vi "Reset Device Core.vi"(8 "error in (no error)":errorcluster, 11 "LS218 in":refnum<class "LS218.lvclass">) -> (0 "error out":errorcluster, 3 "LS218 out":refnum<class "LS218.lvclass">)   [LabVIEW 2013, in "LS218.lvlib" / "LS218.lvclass"]
doc: "Perform reset of device."
uses:
  LS218.lvclass
  CSPP_Core/Actors/CS++DeviceActor/CS++DeviceActor.lvclass
  CSPP_Core/Actors/CS++DeviceActor/CS++DeviceActor.lvclass/CS++DeviceActor.ctl
  LS218.lvclass/LS218.ctl
  CSPP_Core/Actors/CS++DeviceActor/Read ResetWithDefaults.vi
  <instrlib>/Lake Shore Cryotronics 218/Lake Shore Cryotronics 218.lvlib
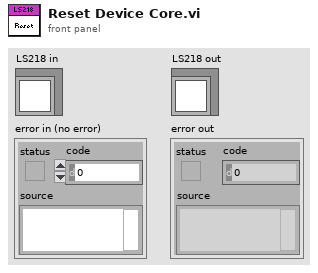
[diagram p1: front panel]
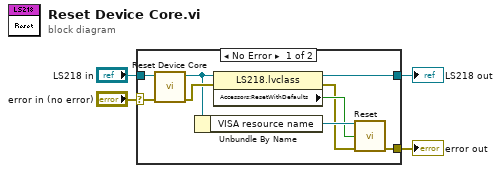
[diagram p0: block diagram]
diagram:
  n1 = case shown="No Error" "error in (no error)" {
    selector: "error in (no error)" -> [w5 w14]
    tunnel: "LS218 in" -> [w13 w15]
    tunnel: [w10 w15] -> w3
    tunnel: [w6 w14] -> w2
    frame No Error {
      n2 = call-parent "Reset Device Core.vi"("error in (no error)"=w5, "CS++DeviceActor in"=w13) -> ("error out"=w9:errorcluster, "CS++DeviceActor out"=w8:refnum<class "LS218.lvclass">)  [unwired: 8 in]
      n3 = Unbundle By Name(w8) -> ("VISA resource name"=w12:refnum<visa-resource-name>)
      n4 = property class="LS218.lvclass"(reference=w8, error in=w9) -> (reference out=w10:refnum<class "LS218.lvclass">, error out=w7:errorcluster, "Accessors:ResetWithDefaults"=w11:bool)
      n5 = call <instrlib>:"Reset.vi"("VISA resource name"=w12, "Reset Defaults (F:Dont Reset)"=w11, "error in (no error)"=w7) -> ("error out"=w6:errorcluster)  [unwired: 11 in, 1 out]
    }
    frame Error {
    }
  }
  "error out" <- w2
  "LS218 out" <- w3
